vi "F5xxx_get_scope_measZ_value.vi"(8 "error in":errorcluster, 11 "VISA in":refnum<visa-resource-name>) -> (0 "error out":errorcluster, 1 "unit":string, 2 "measured value":dbl, 3 "VISA out":refnum<visa-resource-name>)   [LabVIEW 2013]
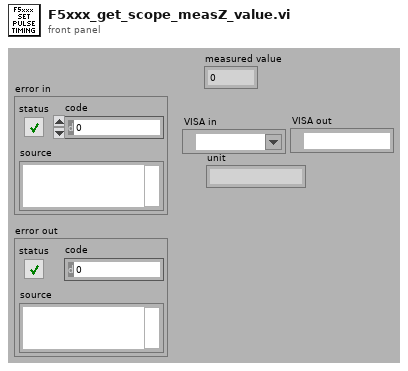
[diagram p1: front panel]
types:
  T1 = cluster{"write buffer":string, "write buffer 2":string}[]
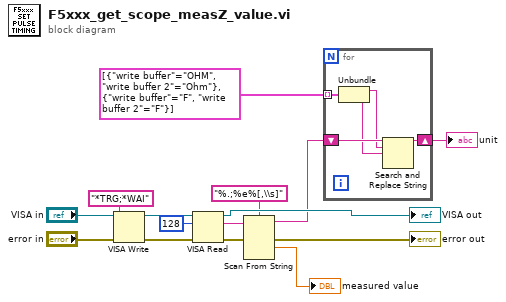
[diagram p0: block diagram]
diagram:
  n1 = VISA Write(VISA resource name="VISA in", write buffer="*TRG;*WAI", error in (no error)="error in") -> (VISA resource name out=w10:refnum<visa-resource-name>, error out=w13:errorcluster)  [unwired: 1 out]
  n2 = VISA Read(VISA resource name=w10, byte count=u32 128, error in (no error)=w13) -> (VISA resource name out=→"VISA out":refnum<visa-resource-name>, read buffer=w5:string, error out=w4:errorcluster)  [unwired: 1 out]
  n3 = Scan From String(format string="%.;%e%[,\\s]", input string=w5, error in=w4) -> (remaining string=w3:string, error out=→"error out":errorcluster, output 1=→"measured value":dbl)  [unwired: 4 in, 1 out]
  n4 = for {
    shift-right: [w19] -> w1
    shift-left: w3 -> [w20]
    tunnel: T1 [{"write buffer"="OHM", "write buffer 2"="Ohm"}, {"write buffer"="F", "write buffer 2"="F"}] -> [w18] mode=indexing
    n5 = Unbundle(w18) -> ("write buffer"=w17:string, "write buffer 2"=w16:string)
    n6 = Search and Replace String(input string=w20, search string=w17, replace string=w16) -> (result string=w19:string)  [unwired: 5 in, 3 out]
  }
  "unit" <- w1
